vi "Acquire Spectrum.vi"(0 "Lens Mode":string="Transmission", 1 "Pass Energy":dbl=150.0, 2 "Region":T1={"fixed_"=0, "highEnergy_"=500.0, "lowEnergy_"=0.0, "centerEnergy_"=0.0, "energyStep_"=10.0, "dwellTime_"=80}, 3 "Detector Region":T2={"firstXChannel_"=1, "lastXChannel_"=1392, "firstYChannel_"=1, "lastYChannel_"=519, "slices_"=519, "adcMode_"=1}, 5 "error in":errorcluster, 14 "Element Set":string) -> (19 "error out":errorcluster)   [LabVIEW 2018]
uses:
  SesWrapper/SesWrapper.lvlib
panel:
  out "kinetic_energy":dbl
  out "energyStep out":dbl
  out "time_ms out":dbl
  out "steps out":i32
  in  "Accumulate":bool
  in  "stop":bool
  out "Analyzer Region out":T1
  out "Detector Region out":T2
  out "Acquisition Data":cluster{"Y":dbl[], "Y":dbl[]}[](graph)
  out "Intensity Graph":dbl[][](graph)
  in  "Spectrum/Image":bool
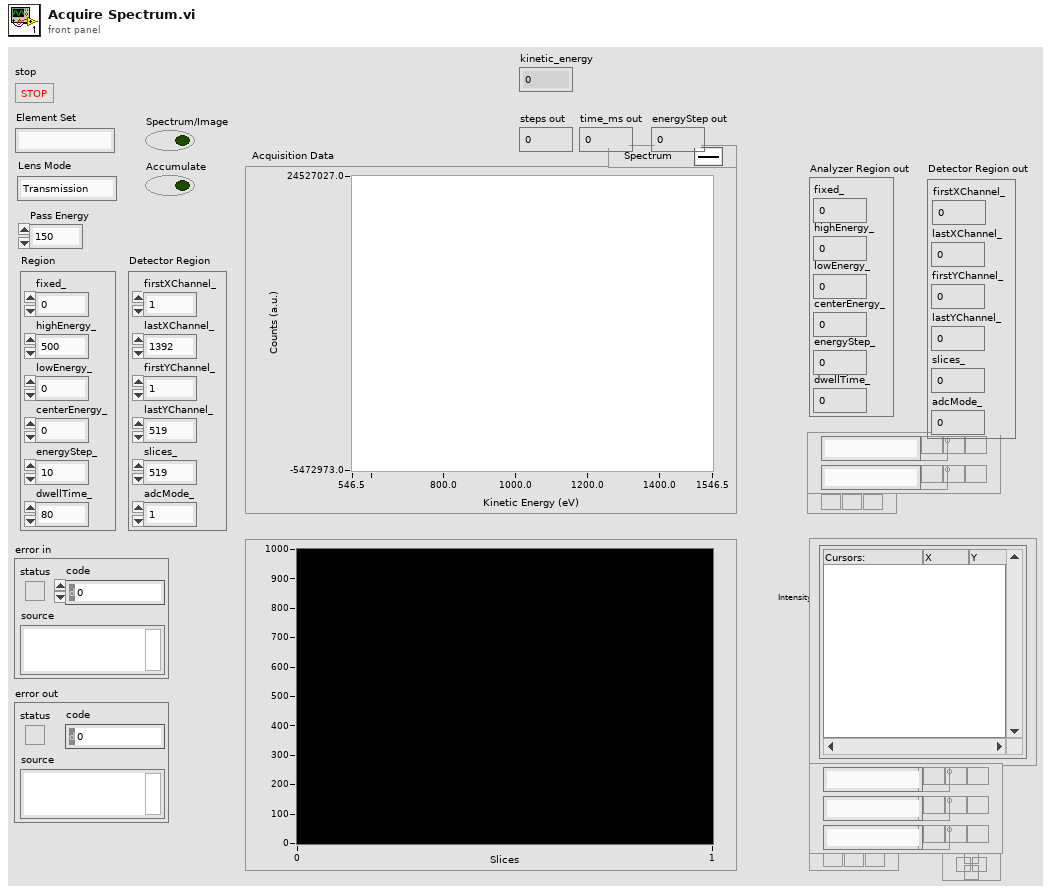
[diagram p1: front panel]
types:
  T1 = cluster{"fixed_":u8, "highEnergy_":dbl, "lowEnergy_":dbl, "centerEnergy_":dbl, "energyStep_":dbl, "dwellTime_":i32}
  T2 = cluster{"firstXChannel_":i32, "lastXChannel_":i32, "firstYChannel_":i32, "lastYChannel_":i32, "slices_":i32, "adcMode_":u8}
  T3 = cluster{"fixed_":u8, "@dummy control@":i8, "@dummy control@":i8, "@dummy control@":i8, "@dummy control@":i8, "@dummy control@":i8, "@dummy control@":i8, "@dummy control@":i8, "highEnergy_":dbl, "lowEnergy_":dbl, "centerEnergy_":dbl, "energyStep_":dbl, "dwellTime_":i32}
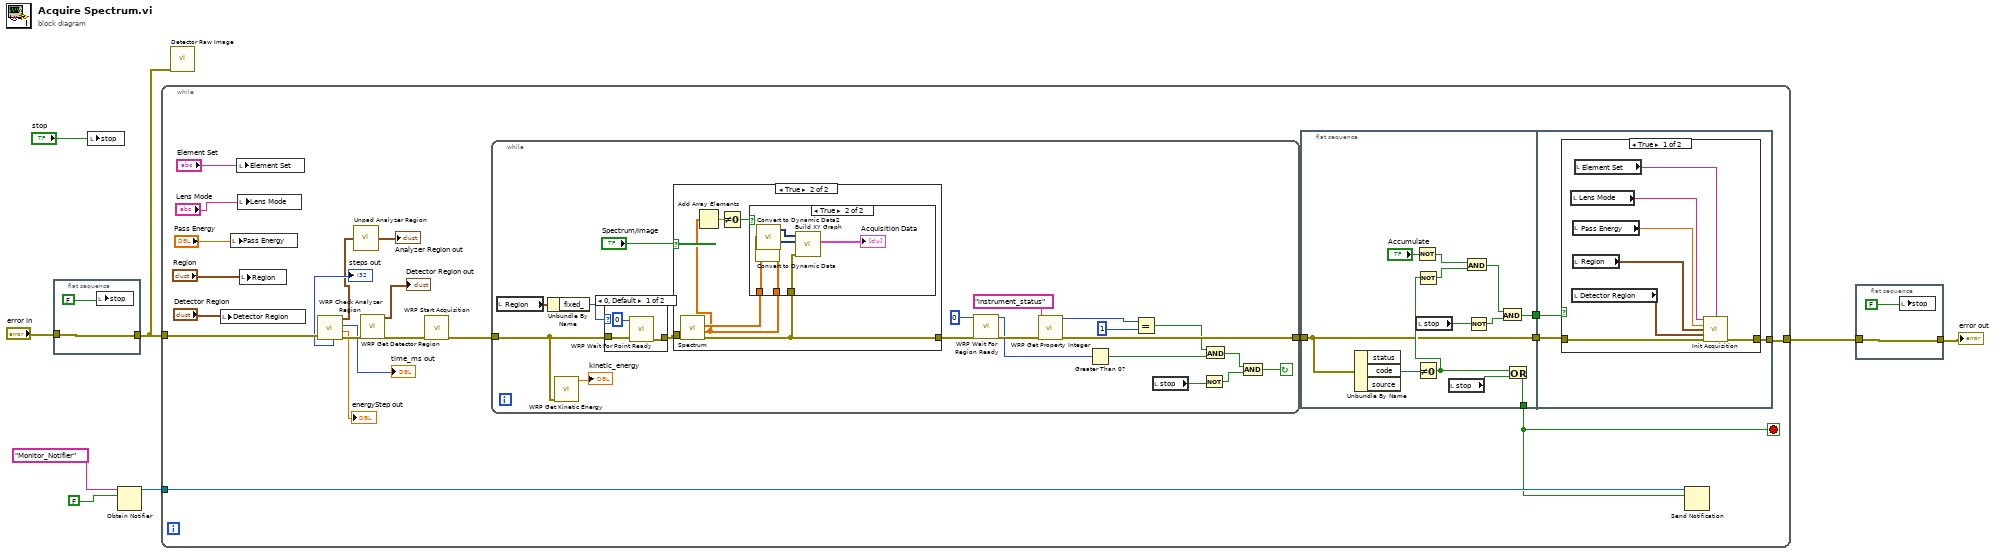
[diagram p0: block diagram]
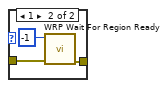
[diagram p3: hidden frame]
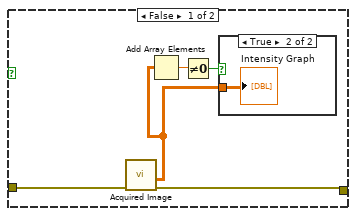
[diagram p4: hidden frame]
diagram:
  n1 = flat-sequence {
    tunnel: "error in" -> [w9]
    tunnel: [w9] -> _
    tunnel: [w9] -> w4
    frame #0 {
      n2 = local write "stop"(FALSE) -> ()
    }
  }
  n3 = local write "stop"("stop") -> ()
  n4 = Obtain Notifier(name (unnamed)="Monitor_Notifier", notification data type=FALSE) -> (notifier out=w1:refnum<notifier>)  [unwired: 2 in, 2 out]
  n5 = while {
    tunnel: [w27] -> w7
    tunnel: w4 -> [w26]
    tunnel: w1 -> [w12]
    stop <- w11 stop-if-true
    n6 = local write "Detector Region"("Detector Region") -> ()
    n7 = local write "Pass Energy"("Pass Energy") -> ()
    n8 = local write "Element Set"("Element Set") -> ()
    n9 = local write "Lens Mode"("Lens Mode") -> ()
    n10 = local write "Region"("Region") -> ()
    n11 = call "WRP Check Analyzer Region.vi"("error in (no error)"=w26) -> ("error out"=w23:errorcluster, "time_ms"=→"energyStep out":dbl, "steps"=→"time_ms out":i32, "analyzerRegion"=w15:T3, "function return"=→"steps out":i32)  [unwired: 5 in, 1 out]
    n12 = call "Unpad Analyzer Region.vi"("Analyzer Region"=w15) -> ("Analyzer Region out"=→"Analyzer Region out":T1)  [unwired: 4 in]
    n13 = call "WRP Get Detector Region.vi"("error in (no error)"=w23) -> ("error out"=w22:errorcluster, "value"=→"Detector Region out":T2)  [unwired: 8 in, 1 out]
    n14 = call "WRP Start Acquisition.vi"("error in (no error)"=w22) -> ("error out"=w13:errorcluster)  [unwired: 9 in, 1 out]
    n15 = while {
      tunnel: w13 -> [w56]
      tunnel: [w67] -> w21
      stop <- w61 continue-if-true
      n16 = local read "Region"() -> (w70:T1)
      n17 = Unbundle By Name(w70) -> ("fixed_"=w71:u8)
      n18 = call "WRP Get Kinetic Energy.vi"("error in (no error)"=w56) -> ("kinetic_energy"=→"kinetic_energy":dbl)  [unwired: 8 in, 2 out]
      n19 = case shown="0, Default" w71 {
        tunnel: [w77 w80] -> w72
        tunnel: w56 -> [w75 w78]
        frame 0, Default {
          n20 = call "WRP Wait For Point Ready.vi"("error in (no error)"=w75, "timeout_ms"=0) -> ("error out"=w77:errorcluster)  [unwired: 8 in, 1 out]
        }
        frame 1 {
          n21 = call "WRP Wait For Region Ready.vi"("error in (no error)"=w78, "timeout_ms"=-1) -> ("error out"=w80:errorcluster)  [unwired: 8 in, 1 out]
        }
      }
      n22 = case shown="True" "Spectrum/Image" {
        tunnel: [w85 w87] -> w64
        tunnel: w72 -> [w81 w88]
        frame False {
          n23 = call "Acquired Image.vi"("error in (no error)"=w81) -> ("error out"=w85:errorcluster, "Image"=w82:dbl[][])  [unwired: 7 in, 2 out]
          n24 = Add Array Elements(numeric array=w82) -> (sum=w83:dbl)
          n25 = Not Equal To 0?(x=w83) -> (x != 0?=w84:bool)
          n26 = case shown="True" w84 {
            tunnel: w82 -> [_ w86]
            frame False {
            }
            frame True {
              "Intensity Graph" <- w86
            }
          }
        }
        frame True {
          n27 = call "Spectrum.vi"("error in (no error)"=w88) -> ("error out"=w87:errorcluster, "Spectrum"=w89:dbl[], "Channel Scale"=w92:dbl[])  [unwired: 7 in, 1 out]
          n28 = Add Array Elements(numeric array=w89) -> (sum=w90:dbl)
          n29 = Not Equal To 0?(x=w90) -> (x != 0?=w91:bool)
          n30 = case shown="True" w91 {
            tunnel: w92 -> [_ w98]
            tunnel: w89 -> [_ w96]
            tunnel: w87 -> [_ w93]
            frame False {
            }
            frame True {
              n31 = call "Convert to Dynamic Data"("Array"=w96) -> ("Dynamic Data Type"=w95:dynamicdata)  [unwired: 3 in]
              n32 = call "Convert to Dynamic Data2"("Array"=w98) -> ("Dynamic Data Type"=w97:dynamicdata)  [unwired: 3 in]
              n33 = call "Build XY Graph"("error in (no error)"=w93, "Y Input"=w95, "X Input"=w97) -> ("XY Graph"=→"Acquisition Data":cluster{"Y":dbl[], "Y":dbl[]}[])  [unwired: 7 in, 1 out]
            }
          }
        }
      }
      n34 = call "WRP Wait For Region Ready.vi"("error in (no error)"=w64, "timeout_ms"=0) -> ("error out"=w68:errorcluster, "function return"=w66:i32)  [unwired: 8 in]
      n35 = call "WRP Get Property Integer.vi"("error in (no error)"=w68, "property"="instrument_status") -> ("error out"=w67:errorcluster, "value"=w57:i32)  [unwired: 6 in, 2 out]
      n36 = Greater Than 0?(x=w66) -> (x > 0?=w63:bool)
      n37 = Equal?(x=w57, y=1) -> (x = y?=w62:bool)
      n38 = local read "stop"() -> (w58:bool)
      n39 = Not(x=w58) -> (.not. x?=w59:bool)
      n40 = And(x=w62, y=w63) -> (x .and. y?=w60:bool)
      n41 = And(x=w60, y=w59) -> (x .and. y?=w61:bool)
    }
    n42 = flat-sequence {
      tunnel: w21 -> [w34]
      tunnel: [w34] -> w20
      tunnel: [w33] -> w19
      tunnel: [w32] -> w11
      tunnel: [w46] -> w27
      tunnel: w20 -> [w45]
      tunnel: w19 -> [w44]
      frame #0 {
        n43 = Unbundle By Name(w34) -> ("code"=w42:i32)  [unwired: 2 out]
        n44 = Not(x="Accumulate") -> (.not. x?=w40:bool)
        n45 = local read "stop"() -> (w35:bool)
        n46 = Not Equal To 0?(x=w42) -> (x != 0?=w38:bool)
        n47 = Not(x=w38) -> (.not. x?=w39:bool)
        n48 = local read "stop"() -> (w43:bool)
        n49 = And(x=w40, y=w39) -> (x .and. y?=w37:bool)
        n50 = Not(x=w35) -> (.not. x?=w36:bool)
        n51 = And(x=w37, y=w36) -> (x .and. y?=w33:bool)
        n52 = Or(x=w38, y=w43) -> (x .or. y?=w32:bool)
      }
      frame #1 {
        n53 = case shown="True" w44 {
          tunnel: [w49 w54] -> w46
          tunnel: w45 -> [w48 w54]
          frame True {
            n54 = local read "Lens Mode"() -> (w53:string)
            n55 = local read "Detector Region"() -> (w50:T2)
            n56 = local read "Pass Energy"() -> (w52:dbl)
            n57 = local read "Region"() -> (w51:T1)
            n58 = local read "Element Set"() -> (w47:string)
            n59 = call "Init Acquisition.vi"("Lens Mode"=w53, "element_set"=w47, "Pass Energy"=w52, "Region"=w51, "Detector Region"=w50, "error in (no error)"=w48) -> ("error out"=w49:errorcluster)  [unwired: 4 in, 5 out]
          }
          frame False {
          }
        }
      }
    }
    n60 = Send Notification(notification=w11, notifier=w12) -> ()  [unwired: 1 in, 2 out]
  }
  n61 = call "Detector Raw Image.vi"("error in (no error)"=w4) -> ()  [unwired: 10 in, 1 out]
  n62 = flat-sequence {
    tunnel: w7 -> [w99]
    tunnel: [w99] -> _
    tunnel: [w99] -> w6
    frame #0 {
      n63 = local write "stop"(FALSE) -> ()
    }
  }
  "error out" <- w6
